vi "hahn echo plus RF.vi"(3 "MW Delay":dbl, 4 "Pulse offset":dbl, 5 "RF Tau":dbl, 6 "MW tau Stop":dbl=1.0 format="%0.2f", 7 "Rabi Frequency":dbl, 8 "MW tau Start":dbl format="%0.2f", 9 "MW tau # samples":i32=128, 10 "No. Instructions":i32, 11 "Optical Pulse":T1(array[cluster])) -> (0 "Pulse Sequence":T1(array[cluster]), 1 "Array":dbl[](array[numeric]))   [LabVIEW 2012]
uses:
  <vilib>/Analysis/1siggen.llb/Ramp Pattern by Samples.vi
  <vilib>/Analysis/NI_AALBase.lvlib
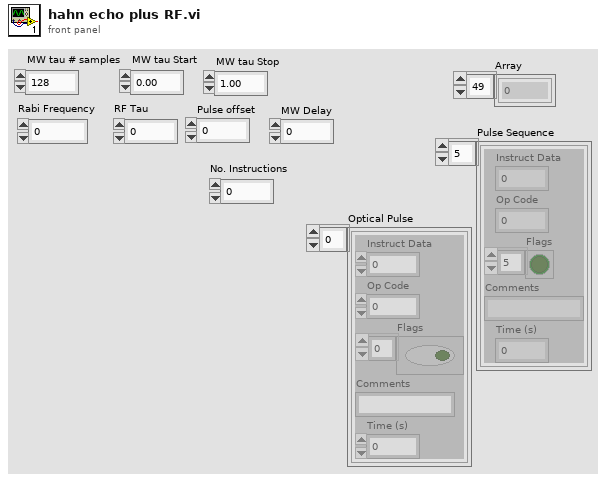
[diagram p1: front panel]
types:
  T1 = cluster{"Instruct Data":i32, "Op Code":i32, "Flags":bool[], "Comments":string, "Time (s)":dbl}[]
  T2 = cluster{"Instruct Data":i32, "Op Code":i32, "Flags":bool[], "Comments":string, "Time (s)":dbl}
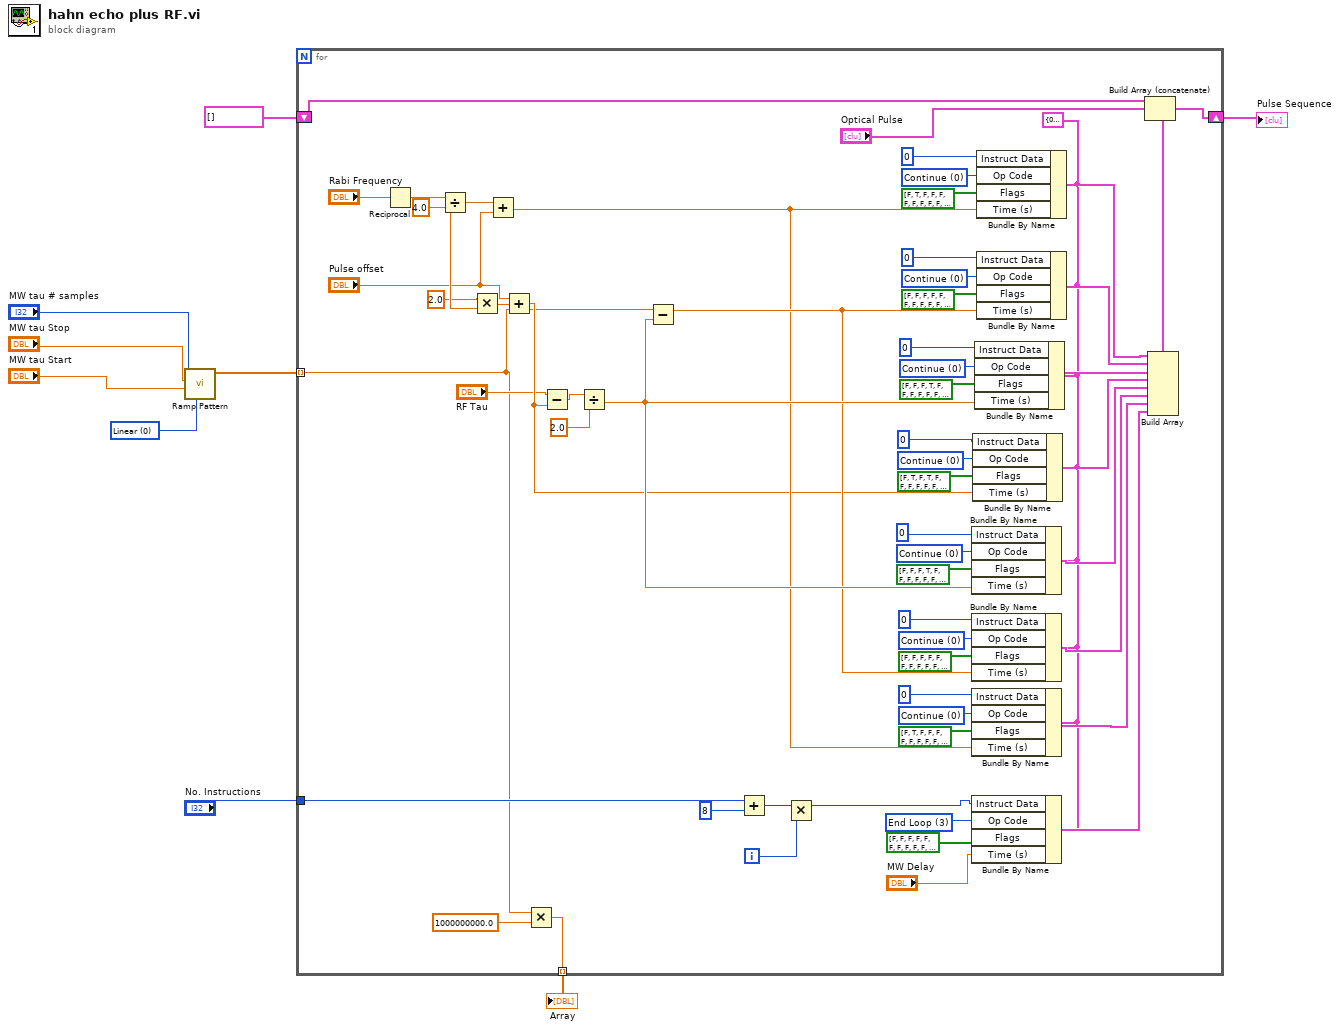
[diagram p0: block diagram]
diagram:
  w5 = u16 0 items=["Linear", "Logarithmic"] ("type")
  n1 = call-poly <vilib>:"Ramp Pattern.vi"("type"=w5, "start"="MW tau Start", "end"="MW tau Stop", "samples"="MW tau # samples") -> ("Ramp Pattern"=w9:dbl[])  [unwired: 6 in, 1 out]
  n2 = for {
    tunnel: w9 -> [w10] mode=indexing
    tunnel: "No. Instructions" -> [w21]
    shift-right: [w15] -> w2
    shift-left: T1 [] -> [w12]
    tunnel: [w13] -> w1 mode=indexing
    i -> [w18]
    w37 = 0 items=["Continue", "Stop", "Loop", "End Loop", "JSR", "RTS", "Branch", "Long Delay", "Wait"] ("Op Code")
    w40 = 0 items=["Continue", "Stop", "Loop", "End Loop", "JSR", "RTS", "Branch", "Long Delay", "Wait"] ("Op Code")
    w47 = 0 items=["Continue", "Stop", "Loop", "End Loop", "JSR", "RTS", "Branch", "Long Delay", "Wait"] ("Op Code")
    w50 = 0 items=["Continue", "Stop", "Loop", "End Loop", "JSR", "RTS", "Branch", "Long Delay", "Wait"] ("Op Code")
    w54 = 0 items=["Continue", "Stop", "Loop", "End Loop", "JSR", "RTS", "Branch", "Long Delay", "Wait"] ("Op Code")
    w57 = 0 items=["Continue", "Stop", "Loop", "End Loop", "JSR", "RTS", "Branch", "Long Delay", "Wait"] ("Op Code")
    w60 = 0 items=["Continue", "Stop", "Loop", "End Loop", "JSR", "RTS", "Branch", "Long Delay", "Wait"] ("Op Code")
    w67 = 3 items=["Continue", "Stop", "Loop", "End Loop", "JSR", "RTS", "Branch", "Long Delay", "Wait"] ("Op Code")
    w24 = T2 {"Instruct Data"=0, "Op Code"=0, "Flags"=[FALSE, FALSE, FALSE, FALSE, FALSE, FALSE, FALSE, FALSE, FALSE, FALSE, FALSE, FALSE, FALSE, FALSE, FALSE, FALSE, FALSE, FALSE, FALSE, FALSE, FALSE, TRUE, TRUE, TRUE], "Comments"="", "Time (s)"=0.01} ("PB Inst 2")
    n3 = Reciprocal(x="Rabi Frequency") -> (1/x=w65:dbl)
    n4 = Divide(x=w65, y=4.0) -> (x/y=w64:dbl)
    n5 = Multiply(x=2.0, y=w64) -> (x*y=w52:dbl)
    n6 = Add(x=w64, y="Pulse offset") -> (x+y=w27:dbl)
    n7 = Add(x="Pulse offset", y=w52) -> (x+y=w26:dbl)
    n8 = Multiply(x=w10, y=1000000000.0) -> (x*y=w13:dbl)
    n9 = Subtract(x="RF Tau", y=w26) -> (x-y=w44:dbl)
    n10 = Divide(x=w44, y=2.0) -> (x/y=w42:dbl)
    n11 = Subtract(x=w10, y=w42) -> (x-y=w35:dbl)
    n12 = Add(x=w21, y=8) -> (x+y=w22:i32)
    n13 = Multiply(x=w22, y=w18) -> (x*y=w19:i32)
    n14 = Bundle By Name(cluster=w24, "Instruct Data"=0, "Op Code"=w47, "Flags"=bool[] [FALSE, FALSE, FALSE, TRUE, FALSE, FALSE, FALSE, FALSE, FALSE, FALSE, FALSE, FALSE, FALSE, FALSE, FALSE, FALSE, FALSE, FALSE, FALSE, FALSE, FALSE, TRUE, TRUE, TRUE], "Time (s)"=w42) -> (w30:T2)
    n15 = Bundle By Name(cluster=w24, "Instruct Data"=0, "Op Code"=w40, "Flags"=bool[] [FALSE, FALSE, FALSE, FALSE, FALSE, FALSE, FALSE, FALSE, FALSE, FALSE, FALSE, FALSE, FALSE, FALSE, FALSE, FALSE, FALSE, FALSE, FALSE, FALSE, FALSE, TRUE, TRUE, TRUE], "Time (s)"=w35) -> (w29:T2)
    n16 = Bundle By Name(cluster=w24, "Instruct Data"=0, "Op Code"=w37, "Flags"=bool[] [FALSE, TRUE, FALSE, FALSE, FALSE, FALSE, FALSE, FALSE, FALSE, FALSE, FALSE, FALSE, FALSE, FALSE, FALSE, FALSE, FALSE, FALSE, FALSE, FALSE, FALSE, TRUE, TRUE, TRUE], "Time (s)"=w27) -> (w28:T2)
    n17 = Bundle By Name(cluster=w24, "Instruct Data"=w19, "Op Code"=w67, "Flags"=bool[] [FALSE, FALSE, FALSE, FALSE, FALSE, FALSE, FALSE, FALSE, FALSE, FALSE, FALSE, FALSE, FALSE, FALSE, FALSE, FALSE, FALSE, FALSE, FALSE, FALSE, FALSE, TRUE, TRUE, TRUE], "Time (s)"="MW Delay") -> (w25:T2)
    n18 = Bundle By Name(cluster=w24, "Instruct Data"=0, "Op Code"=w50, "Flags"=bool[] [FALSE, TRUE, FALSE, TRUE, FALSE, FALSE, FALSE, FALSE, FALSE, FALSE, FALSE, FALSE, FALSE, FALSE, FALSE, FALSE, FALSE, FALSE, FALSE, FALSE, FALSE, TRUE, TRUE, TRUE], "Time (s)"=w26) -> (w31:T2)
    n19 = Bundle By Name(cluster=w24, "Instruct Data"=0, "Op Code"=w54, "Flags"=bool[] [FALSE, FALSE, FALSE, TRUE, FALSE, FALSE, FALSE, FALSE, FALSE, FALSE, FALSE, FALSE, FALSE, FALSE, FALSE, FALSE, FALSE, FALSE, FALSE, FALSE, FALSE, TRUE, TRUE, TRUE], "Time (s)"=w42) -> (w32:T2)
    n20 = Bundle By Name(cluster=w24, "Instruct Data"=0, "Op Code"=w60, "Flags"=bool[] [FALSE, TRUE, FALSE, FALSE, FALSE, FALSE, FALSE, FALSE, FALSE, FALSE, FALSE, FALSE, FALSE, FALSE, FALSE, FALSE, FALSE, FALSE, FALSE, FALSE, FALSE, TRUE, TRUE, TRUE], "Time (s)"=w27) -> (w34:T2)
    n21 = Bundle By Name(cluster=w24, "Instruct Data"=0, "Op Code"=w57, "Flags"=bool[] [FALSE, FALSE, FALSE, FALSE, FALSE, FALSE, FALSE, FALSE, FALSE, FALSE, FALSE, FALSE, FALSE, FALSE, FALSE, FALSE, FALSE, FALSE, FALSE, FALSE, FALSE, TRUE, TRUE, TRUE], "Time (s)"=w35) -> (w33:T2)
    n22 = Build Array(w34, w33, w32, w31, w30, w29, w28, w25) -> (w17:T1)
    n23 = Build Array (concatenate)(w12, "Optical Pulse", w17) -> (w15:T1)
  }
  "Pulse Sequence" <- w2
  "Array" <- w1
